vi "set control position.vi"(8 "error in (no error)":errorcluster, 9 "ignore caption & label? (T)":bool=TRUE, 10 "Position":T1, 11 "Control in":refnum<class "Control.lvclass">) -> (0 "error out":errorcluster, 3 "Control out":refnum<class "Control.lvclass">)   [LabVIEW 2010, in "Control.lvclass"]
uses:
  Control.lvclass
  <vilib>/Utility/miscctls.llb/LVPositionTypeDef.ctl
  Control.lvclass/Control.ctl
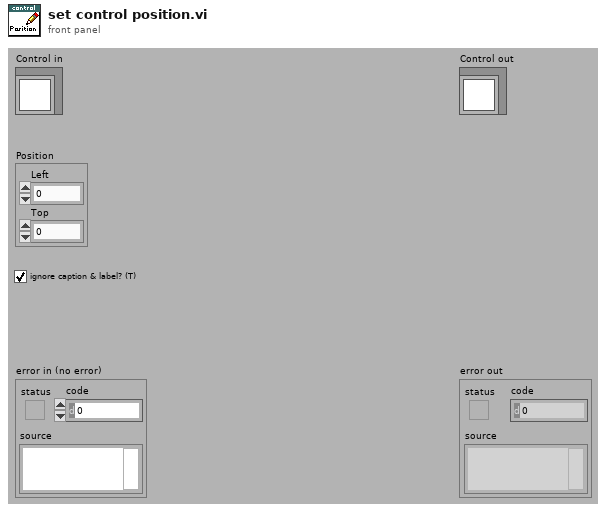
[diagram p1: front panel]
types:
  T1 = typedef "LVPositionTypeDef.ctl" = cluster{"Left":i32, "Top":i32}
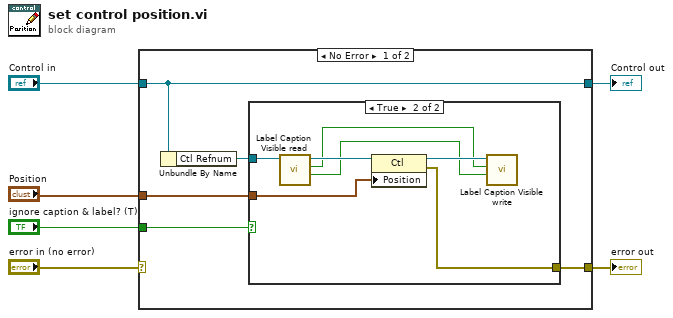
[diagram p0: block diagram]
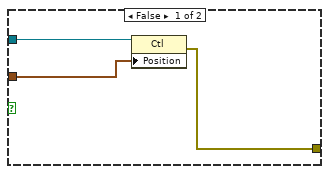
[diagram p2: hidden frame]
diagram:
  n1 = case shown="No Error" "error in (no error)" {
    selector: "error in (no error)" -> [_ w23]
    tunnel: [w9 w23] -> w5
    tunnel: [w11 w22] -> w3
    tunnel: "Control in" -> [w11 w22]
    tunnel: "Position" -> [w8 _]
    tunnel: "ignore caption & label? (T)" -> [w7 _]
    frame No Error {
      n2 = Unbundle By Name(w11) -> ("Ctl Refnum"=w10:refnum<vi>)
      n3 = case shown="True" w7 {
        tunnel: w10 -> [w14 w19]
        tunnel: [w13 w21] -> w9
        tunnel: w8 -> [w12 w20]
        frame False {
          n4 = property class="Ctl"(reference=w14, "Position"=w12) -> (error out=w13:errorcluster)  [unwired: 1 in, 1 out]
        }
        frame True {
          n5 = call "Label Caption Visible read.vi"("Ctl Refnum in"=w19) -> ("Caption.Visible"=w15:bool, "Label.Visible"=w16:bool, "Ctl Refnum out"=w18:refnum<vi>)  [unwired: 6 in]
          n6 = property class="Ctl"(reference=w18, "Position"=w20) -> (reference out=w17:refnum<vi>, error out=w21:errorcluster)  [unwired: 1 in]
          n7 = call "Label Caption Visible write.vi"("Caption.Visible"=w15, "Label.Visible"=w16, "Ctl Refnum in"=w17) -> ()  [unwired: 6 in, 1 out]
        }
      }
    }
    frame Error {
    }
  }
  "error out" <- w5
  "Control out" <- w3
